vi "Simple State Machine (Generate random number's for each click).vi"() -> ()   [LabVIEW 2017]
panel:
  in  "Generate":bool
  in  "stop":bool
  out "Numeric":dbl
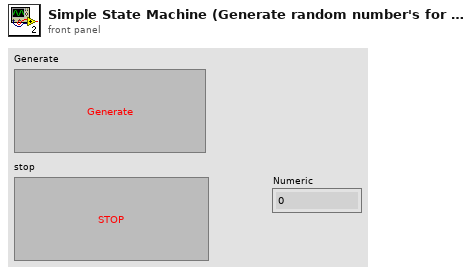
[diagram p1: front panel]
types:
  T1 = enum16{"Initialize", "Main idle / Wait for event", "Stop"}
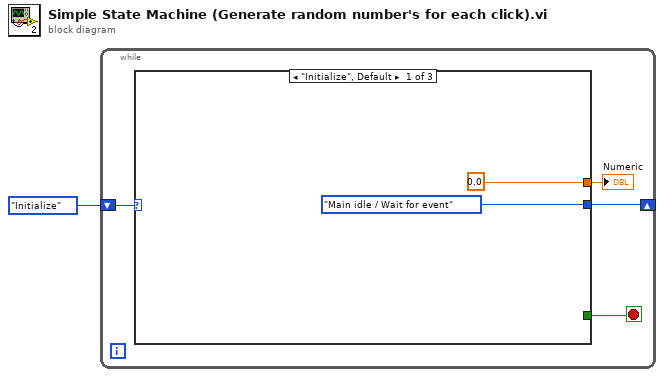
[diagram p0: block diagram]
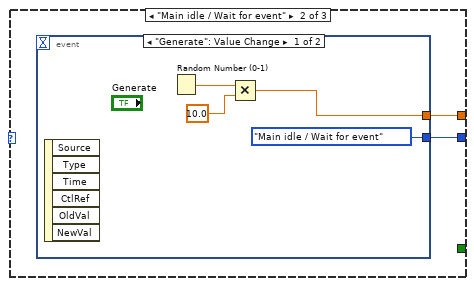
[diagram p2: hidden frame]
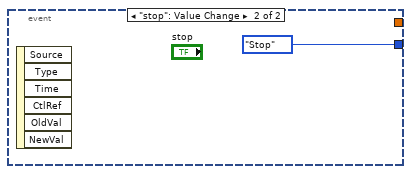
[diagram p3: hidden frame]
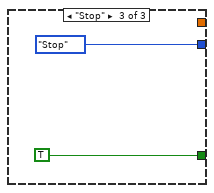
[diagram p4: hidden frame]
diagram:
  n1 = while {
    shift-right: [w4] -> _
    shift-left: T1."Initialize" ("Enum") -> [w5]
    stop <- w2 stop-if-true
    n2 = case shown="\"Initialize\", Default" w5 {
      tunnel: [T1."Main idle / Wait for event" ("Enum 2") w9 T1."Stop" ("Enum 2")] -> w4
      tunnel: [0.0 w8 _] -> w3
      tunnel: [_ _ TRUE] -> w2
      frame "Initialize", Default {
      }
      frame "Main idle / Wait for event" {
        n3 = event shown="[0] \"Generate\": Value Change" {
          selector: _ -> [_ _]
          dyn-events: _ -> [_ _]
          timeout: _ -> [_ _]
          tunnel: [T1."Main idle / Wait for event" ("Enum 2") T1."Stop" ("Enum 2")] -> w9
          tunnel: [w10 _] -> w8
          event "Generate": Value Change {
            n4 = event-data() -> ()  [unwired: 1 in, 6 out]
            n5 = Random Number (0-1)() -> (number: 0 to 1=w12:dbl)
            n6 = Multiply(x=w12, y=10.0) -> (x*y=w10:dbl)
          }
          event "stop": Value Change {
            n7 = event-data() -> ()  [unwired: 1 in, 6 out]
          }
        }
      }
      frame "Stop" {
      }
    }
    "Numeric" <- w3
  }
